vi "HumiditySensorHost.vi"() -> (18 "Waveform Chart":cluster{dbl, dbl}(graph), 20 "Temperature (°C)":fxp<+,16,7> format="%#_3g", 22 "Humidity (%)":fxp<+/-,18,8> format="%#_3g", 25 "Humidity sensor Communication":errorcluster, 27 "FPGA Error":errorcluster)   [LabVIEW 2016]
doc: "Host VI for getting humidity and temperature data from FPGA VI of DHT 22 sensor.\nHumidity signal is relative humidity in percentage. Temperature signal gives temperature in degrees Celsius."
uses:
  <vilib>/userdefined/High Color/nirio_resource_hc.ctl
  <vilib>/FPGAPlugInAG/myRIO-1900/niLvFpga_Open_myRIO-1900.vi
  <vilib>/FPGAPlugInAG/myRIO-1900/niLvFpga_Run_myRIO-1900.vi
  <vilib>/Utility/error.llb/Error Cluster From Error Code.vi
  <vilib>/rvi/errors/niLvFpgaAdjustHostInterfaceError.vi
  <vilib>/FPGAPlugInAG/myRIO-1900/niLvFpga_Close_myRIO-1900.vi
  <vilib>/rvi/interface/nirviOpenFPGA/nirviOpenFPGA.xnode
  FPGA Bitfiles/WeatherStationPr_FPGATarget_HumiditySensorIn_HuBObqjwKeQ.lvbitx
  <vilib>/rvi/interface/nirviMethod/nirviMethod.xnode
  <vilib>/rvi/interface/nirviReadWriteControl/nirviReadWriteControl.xnode
  <vilib>/rvi/interface/nirviCloseFPGA/nirviCloseFPGA.xnode
  NiFpgaLv.dll
panel:
  in  "stop":bool
  in  "stop 2":bool
  # "Humidity and Temperature Readings"
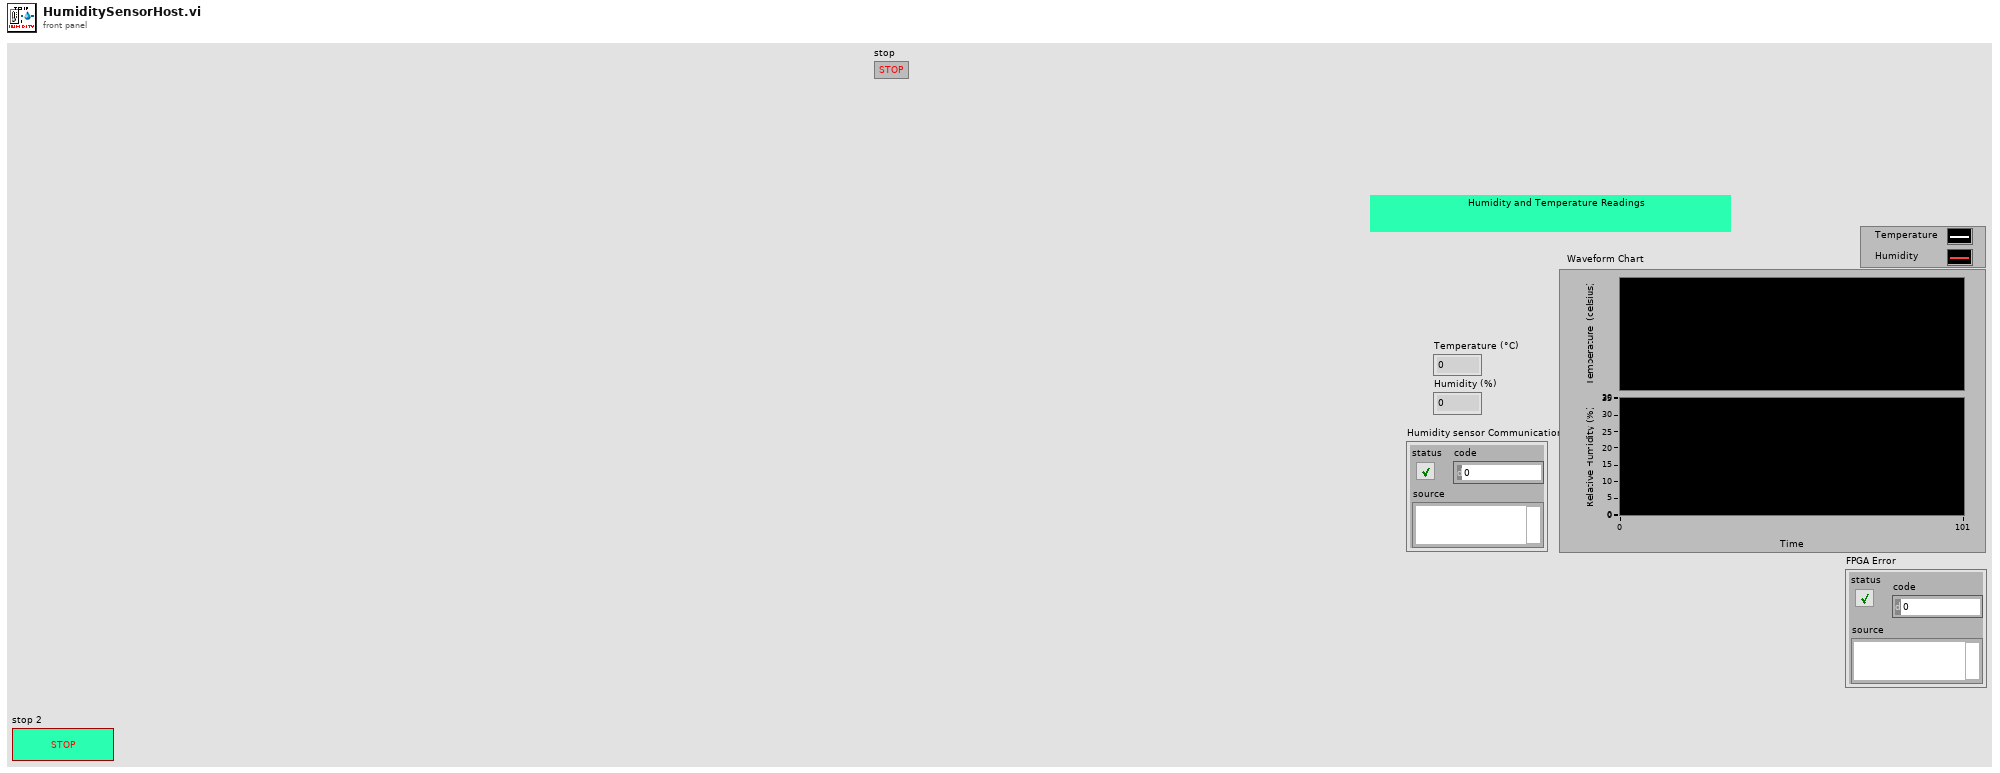
[diagram p1: front panel]
types:
  T1 = typedef "nirio_resource_hc.ctl" = tag
  T2 = cluster{"Temperature (°C)":fxp<+,16,7>, "Humidity (%)":fxp<+/-,18,8>}
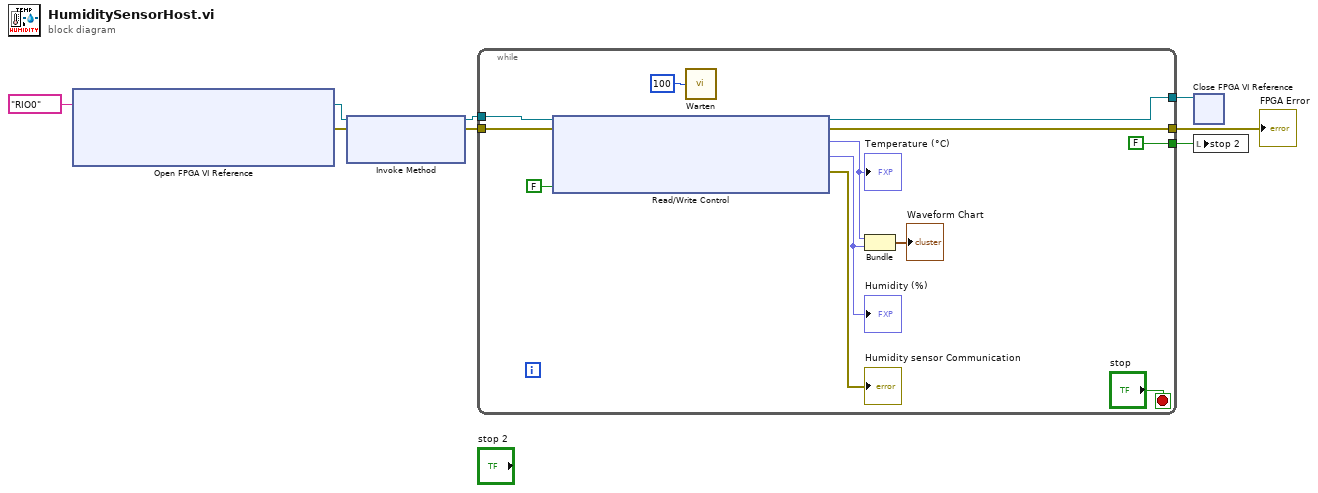
[diagram p0: block diagram]
diagram:
  n1 = xnode "Open FPGA VI Reference"("resource name"=T1 "RIO0") -> ("FPGA VI Reference Out"=w5:refnum<k20>, "error out"=w4:errorcluster)  [unwired: 1 in]
  n2 = xnode "Invoke Method"("FPGA VI Reference In"=w5, "error in"=w4) -> ("FPGA VI Reference Out"=w3:refnum<k20>, "error out"=w2:errorcluster)  [unwired: 1 in]
  n3 = while {
    tunnel: [w15] -> w8
    tunnel: [w13] -> w1
    tunnel: [FALSE] -> w7
    tunnel: w3 -> [w11]
    tunnel: w2 -> [w10]
    stop <- "stop" stop-if-true
    n4 = xnode "Read/Write Control"("FPGA VI Reference In"=w11, "error in"=w10, "STOP Reading Inputs"=FALSE ("Warten bis beendet (F)")) -> ("FPGA VI Reference Out"=w13:refnum<k20>, "error out"=w15:errorcluster, "Temperature (°C)"=w18:fxp<+,16,7>, "Humidity (%)"=w19:fxp<+/-,18,8>, "error out"=→"Humidity sensor Communication":errorcluster)
    "Temperature (°C)" <- w18
    "Humidity (%)" <- w19
    n5 = call "Warten"("Count(mSec)"=u32 100) -> ()  [unwired: 1 out]
    n6 = Bundle("Temperature (°C)"=w18, "Humidity (%)"=w19) -> (→"Waveform Chart":T2)  [unwired: 1 in]
  }
  "FPGA Error" <- w8
  n7 = xnode "Close FPGA VI Reference"("FPGA VI Reference In"=w1) -> ()  [unwired: 1 in, 1 out]
  n8 = local write "stop 2"(w7) -> ()
